vi "VI Tree.vi"   [LabVIEW 2015, in "Keithley 2450.lvlib"]
doc: "This is the instrument driver for the Keithley 2400 Series SourceMeter. The VI Tree displays all the user-callable VIs of the instrument driver in an organized table."
uses:
  <instrlib>/Keithley 2450/Keithley 2450.lvlib
panel:
  # "SEE DIAGRAM\nFOR VI TREE."
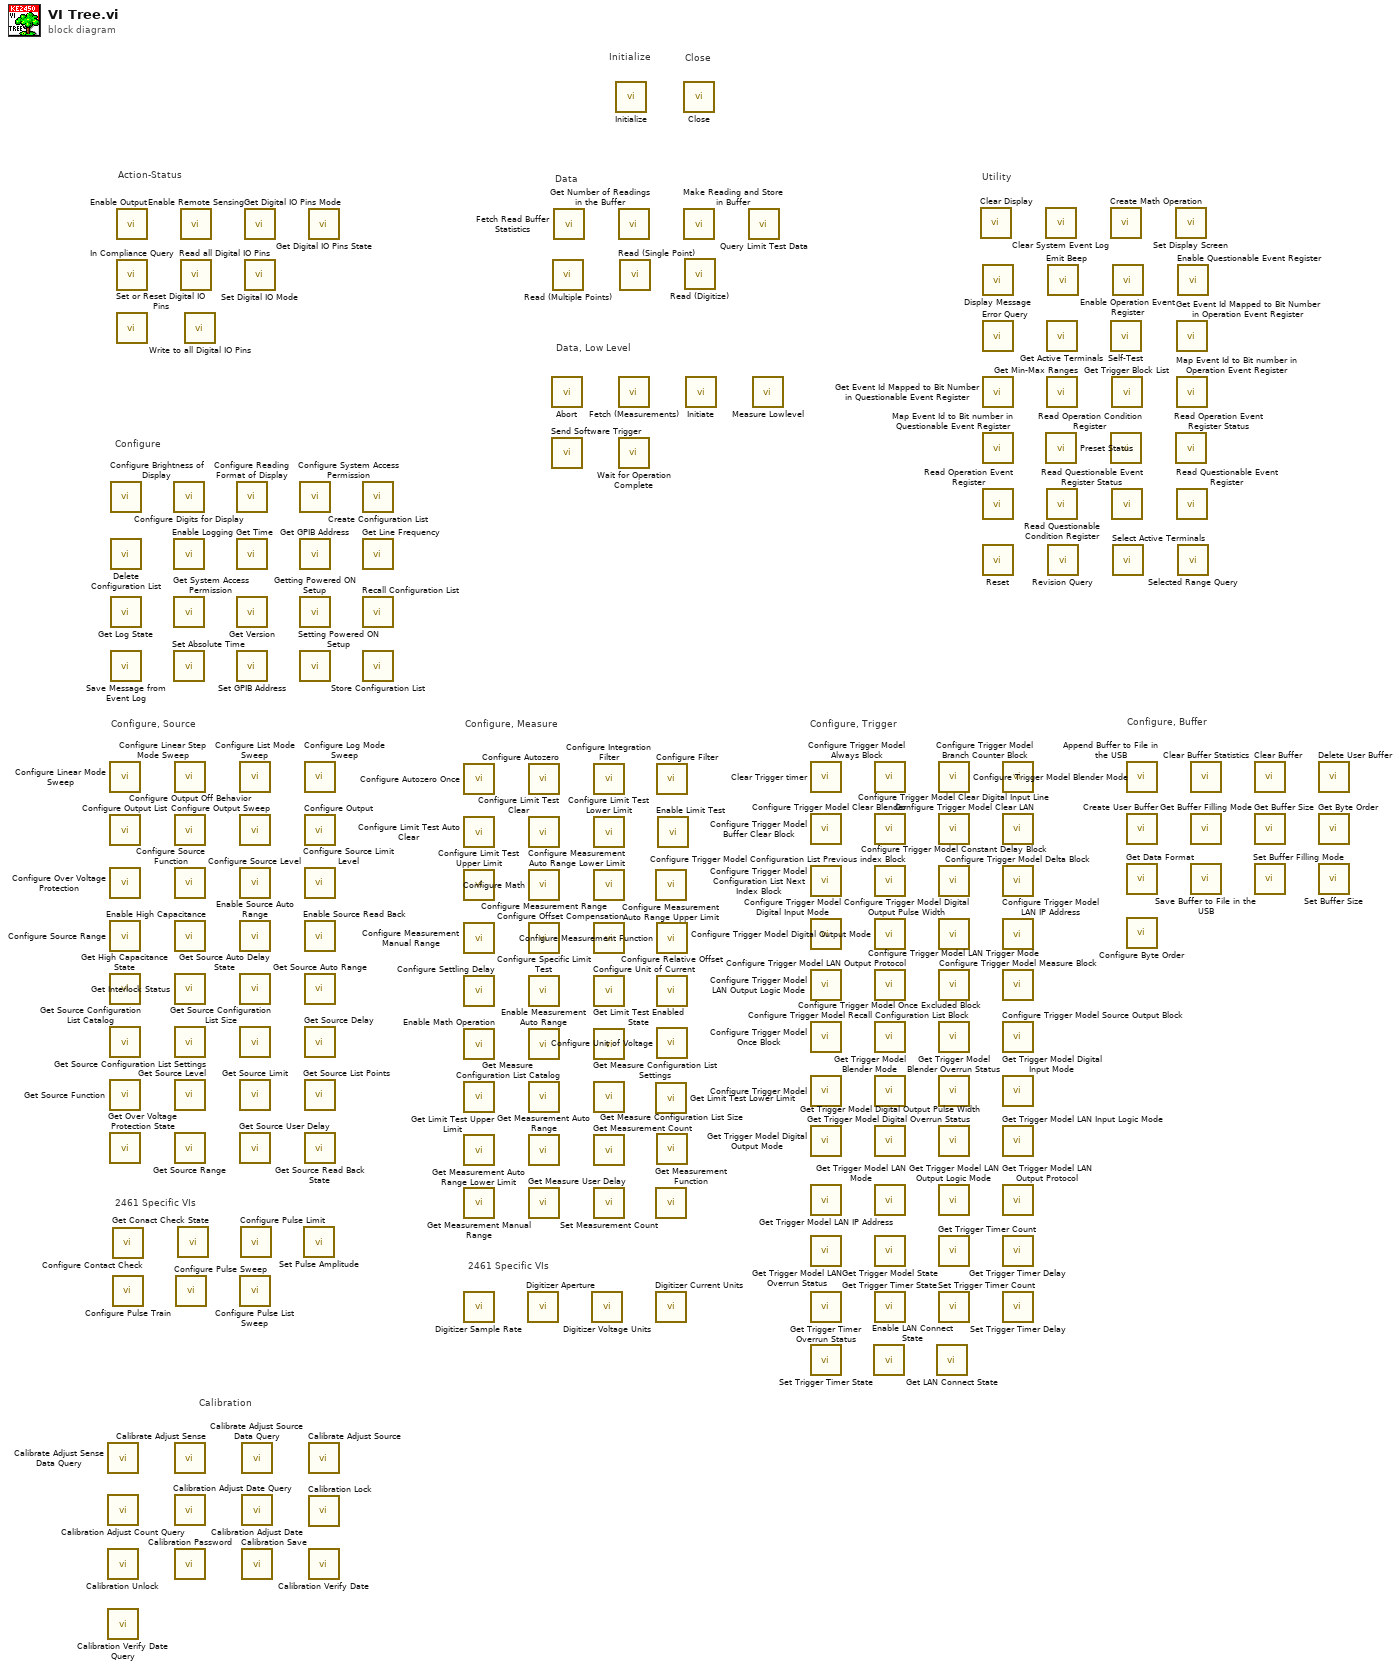
[diagram p0: block diagram]
diagram:
  # "2461 Specific VIs"
  # "Calibration"
  # "2461 Specific VIs"
  # "Configure, Buffer"
  # "Configure, Trigger"
  # "Configure, Measure"
  # "Configure, Source"
  # "Configure"
  # "Utility"
  # "Data, Low Level"
  # "Data"
  # "Action-Status"
  # "Close"
  # "Initialize"
  n1 = call <instrlib>:"Calibrate Adjust Sense Data Query.vi"() -> ()  [unwired: 9 in, 3 out]
  n2 = call <instrlib>:"Calibration Adjust Count Query.vi"() -> ()  [unwired: 9 in, 3 out]
  n3 = call <instrlib>:"Calibration Unlock.vi"() -> ()  [unwired: 10 in, 2 out]
  n4 = call <instrlib>:"Calibration Verify Date Query.vi"() -> ()  [unwired: 9 in, 3 out]
  n5 = call <instrlib>:"Configure Linear Mode Sweep.vi"() -> ()  [unwired: 18 in, 2 out]
  n6 = call <instrlib>:"Configure Output List.vi"() -> ()  [unwired: 10 in, 2 out]
  n7 = call <instrlib>:"Configure Over Voltage Protection.vi"() -> ()  [unwired: 10 in, 2 out]
  n8 = call <instrlib>:"Configure Source Range.vi"() -> ()  [unwired: 10 in, 2 out]
  n9 = call <instrlib>:"Get High Capacitance State.vi"() -> ()  [unwired: 8 in, 4 out]
  n10 = call <instrlib>:"Get Source Configuration List Catalog.vi"() -> ()  [unwired: 9 in, 3 out]
  n11 = call <instrlib>:"Get Source Function.vi"() -> ()  [unwired: 9 in, 3 out]
  n12 = call <instrlib>:"Get Over Voltage Protection State.vi"() -> ()  [unwired: 9 in, 3 out]
  n13 = call <instrlib>:"Configure Brightness of Display.vi"() -> ()  [unwired: 10 in, 2 out]
  n14 = call <instrlib>:"Delete Configuration List.vi"() -> ()  [unwired: 18 in, 2 out]
  n15 = call <instrlib>:"Get Log State.vi"() -> ()  [unwired: 9 in, 3 out]
  n16 = call <instrlib>:"Save Message from Event Log.vi"() -> ()  [unwired: 10 in, 2 out]
  n17 = call <instrlib>:"Configure Contact Check.vi"() -> ()  [unwired: 10 in, 2 out]
  n18 = call <instrlib>:"Configure Pulse Train.vi"() -> ()  [unwired: 18 in, 2 out]
  n19 = call <instrlib>:"Enable Output.vi"() -> ()  [unwired: 10 in, 2 out]
  n20 = call <instrlib>:"In Compliance Query.vi"() -> ()  [unwired: 8 in, 4 out]
  n21 = call <instrlib>:"Set or Reset Digital IO Pins.vi"() -> ()  [unwired: 10 in, 2 out]
  n22 = call <instrlib>:"Configure Digits for Display.vi"() -> ()  [unwired: 10 in, 2 out]
  n23 = call <instrlib>:"Enable Logging.vi"() -> ()  [unwired: 10 in, 2 out]
  n24 = call <instrlib>:"Get System Access Permission.vi"() -> ()  [unwired: 9 in, 3 out]
  n25 = call <instrlib>:"Set Absolute Time.vi"() -> ()  [unwired: 10 in, 2 out]
  n26 = call <instrlib>:"Configure Linear Step Mode Sweep.vi"() -> ()  [unwired: 18 in, 2 out]
  n27 = call <instrlib>:"Configure Output Off Behavior.vi"() -> ()  [unwired: 10 in, 2 out]
  n28 = call <instrlib>:"Configure Source Function.vi"() -> ()  [unwired: 10 in, 2 out]
  n29 = call <instrlib>:"Enable High Capacitance.vi"() -> ()  [unwired: 10 in, 2 out]
  n30 = call <instrlib>:"Get Interlock Status.vi"() -> ()  [unwired: 9 in, 3 out]
  n31 = call <instrlib>:"Get Source Configuration List Settings.vi"() -> ()  [unwired: 17 in, 3 out]
  n32 = call <instrlib>:"Get Source Level.vi"() -> ()  [unwired: 8 in, 4 out]
  n33 = call <instrlib>:"Get Source Range.vi"() -> ()  [unwired: 8 in, 4 out]
  n34 = call <instrlib>:"Calibrate Adjust Sense.vi"() -> ()  [unwired: 10 in, 2 out]
  n35 = call <instrlib>:"Calibration Adjust Date Query.vi"() -> ()  [unwired: 9 in, 3 out]
  n36 = call <instrlib>:"Calibration Password.vi"() -> ()  [unwired: 10 in, 2 out]
  n37 = call <instrlib>:"Configure Pulse Sweep.vi"() -> ()  [unwired: 18 in, 2 out]
  n38 = call <instrlib>:"Get Conact Check State.vi"() -> ()  [unwired: 6 in, 6 out]
  n39 = call <instrlib>:"Enable Remote Sensing.vi"() -> ()  [unwired: 10 in, 2 out]
  n40 = call <instrlib>:"Read all Digital IO Pins.vi"() -> ()  [unwired: 9 in, 3 out]
  n41 = call <instrlib>:"Write to all Digital IO Pins.vi"() -> ()  [unwired: 10 in, 2 out]
  n42 = call <instrlib>:"Configure Reading Format of Display.vi"() -> ()  [unwired: 10 in, 2 out]
  n43 = call <instrlib>:"Get Time.vi"() -> ()  [unwired: 8 in, 4 out]
  n44 = call <instrlib>:"Get Version.vi"() -> ()  [unwired: 9 in, 3 out]
  n45 = call <instrlib>:"Set GPIB Address.vi"() -> ()  [unwired: 10 in, 2 out]
  n46 = call <instrlib>:"Configure List Mode Sweep.vi"() -> ()  [unwired: 14 in, 2 out]
  n47 = call <instrlib>:"Configure Output Sweep.vi"() -> ()  [unwired: 14 in, 2 out]
  n48 = call <instrlib>:"Configure Source Level.vi"() -> ()  [unwired: 10 in, 2 out]
  n49 = call <instrlib>:"Enable Source Auto Range.vi"() -> ()  [unwired: 10 in, 2 out]
  n50 = call <instrlib>:"Get Source Auto Delay State.vi"() -> ()  [unwired: 9 in, 3 out]
  n51 = call <instrlib>:"Get Source Configuration List Size.vi"() -> ()  [unwired: 9 in, 3 out]
  n52 = call <instrlib>:"Get Source Limit.vi"() -> ()  [unwired: 8 in, 4 out]
  n53 = call <instrlib>:"Get Source User Delay.vi"() -> ()  [unwired: 9 in, 3 out]
  n54 = call <instrlib>:"Configure Pulse List Sweep.vi"() -> ()  [unwired: 18 in, 2 out]
  n55 = call <instrlib>:"Configure Pulse Limit.vi"() -> ()  [unwired: 10 in, 2 out]
  n56 = call <instrlib>:"Calibrate Adjust Source Data Query.vi"() -> ()  [unwired: 9 in, 3 out]
  n57 = call <instrlib>:"Calibration Adjust Date.vi"() -> ()  [unwired: 10 in, 2 out]
  n58 = call <instrlib>:"Calibration Save.vi"() -> ()  [unwired: 10 in, 2 out]
  n59 = call <instrlib>:"Get Digital IO Pins Mode.vi"() -> ()  [unwired: 9 in, 3 out]
  n60 = call <instrlib>:"Set Digital IO Mode.vi"() -> ()  [unwired: 10 in, 2 out]
  n61 = call <instrlib>:"Configure System Access Permission.vi"() -> ()  [unwired: 10 in, 2 out]
  n62 = call <instrlib>:"Get GPIB Address.vi"() -> ()  [unwired: 9 in, 3 out]
  n63 = call <instrlib>:"Getting Powered ON Setup.vi"() -> ()  [unwired: 9 in, 3 out]
  n64 = call <instrlib>:"Setting Powered ON Setup.vi"() -> ()  [unwired: 10 in, 2 out]
  n65 = call <instrlib>:"Set Pulse Amplitude.vi"() -> ()  [unwired: 10 in, 2 out]
  n66 = call <instrlib>:"Configure Log Mode Sweep.vi"() -> ()  [unwired: 18 in, 2 out]
  n67 = call <instrlib>:"Configure Output.vi"() -> ()  [unwired: 14 in, 2 out]
  n68 = call <instrlib>:"Configure Source Limit Level.vi"() -> ()  [unwired: 10 in, 2 out]
  n69 = call <instrlib>:"Enable Source Read Back.vi"() -> ()  [unwired: 10 in, 2 out]
  n70 = call <instrlib>:"Get Source Auto Range.vi"() -> ()  [unwired: 8 in, 4 out]
  n71 = call <instrlib>:"Get Source Delay.vi"() -> ()  [unwired: 9 in, 3 out]
  n72 = call <instrlib>:"Get Source List Points.vi"() -> ()  [unwired: 8 in, 4 out]
  n73 = call <instrlib>:"Get Source Read Back State.vi"() -> ()  [unwired: 8 in, 4 out]
  n74 = call <instrlib>:"Get Digital IO Pins State.vi"() -> ()  [unwired: 9 in, 3 out]
  n75 = call <instrlib>:"Calibrate Adjust Source.vi"() -> ()  [unwired: 10 in, 2 out]
  n76 = call <instrlib>:"Calibration Lock.vi"() -> ()  [unwired: 10 in, 2 out]
  n77 = call <instrlib>:"Calibration Verify Date.vi"() -> ()  [unwired: 10 in, 2 out]
  n78 = call <instrlib>:"Create Configuration List.vi"() -> ()  [unwired: 10 in, 2 out]
  n79 = call <instrlib>:"Get Line Frequency.vi"() -> ()  [unwired: 9 in, 3 out]
  n80 = call <instrlib>:"Recall Configuration List.vi"() -> ()  [unwired: 18 in, 2 out]
  n81 = call <instrlib>:"Store Configuration List.vi"() -> ()  [unwired: 18 in, 2 out]
  n82 = call <instrlib>:"Configure Autozero Once.vi"() -> ()  [unwired: 10 in, 2 out]
  n83 = call <instrlib>:"Configure Limit Test Auto Clear.vi"() -> ()  [unwired: 14 in, 2 out]
  n84 = call <instrlib>:"Configure Limit Test Upper Limit.vi"() -> ()  [unwired: 14 in, 2 out]
  n85 = call <instrlib>:"Configure Measurement Manual Range.vi"() -> ()  [unwired: 10 in, 2 out]
  n86 = call <instrlib>:"Configure Settling Delay.vi"() -> ()  [unwired: 10 in, 2 out]
  n87 = call <instrlib>:"Enable Math Operation.vi"() -> ()  [unwired: 10 in, 2 out]
  n88 = call <instrlib>:"Get Limit Test Upper Limit.vi"() -> ()  [unwired: 13 in, 3 out]
  n89 = call <instrlib>:"Get Measurement Auto Range Lower Limit.vi"() -> ()  [unwired: 11 in, 5 out]
  n90 = call <instrlib>:"Get Measurement Manual Range.vi"() -> ()  [unwired: 11 in, 5 out]
  n91 = call <instrlib>:"Digitizer Sample Rate.vi"() -> ()  [unwired: 10 in, 2 out]
  n92 = call <instrlib>:"Digitizer Aperture.vi"() -> ()  [unwired: 14 in, 2 out]
  n93 = call <instrlib>:"Configure Autozero.vi"() -> ()  [unwired: 10 in, 2 out]
  n94 = call <instrlib>:"Configure Limit Test Clear.vi"() -> ()  [unwired: 14 in, 2 out]
  n95 = call <instrlib>:"Configure Math.vi"() -> ()  [unwired: 18 in, 2 out]
  n96 = call <instrlib>:"Configure Measurement Range.vi"() -> ()  [unwired: 10 in, 2 out]
  n97 = call <instrlib>:"Configure Specific Limit Test.vi"() -> ()  [unwired: 14 in, 2 out]
  n98 = call <instrlib>:"Enable Measurement Auto Range.vi"() -> ()  [unwired: 10 in, 2 out]
  n99 = call <instrlib>:"Get Measure Configuration List Catalog.vi"() -> ()  [unwired: 9 in, 3 out]
  n100 = call <instrlib>:"Get Measurement Auto Range.vi"() -> ()  [unwired: 11 in, 5 out]
  n101 = call <instrlib>:"Get Measure User Delay.vi"() -> ()  [unwired: 9 in, 3 out]
  n102 = call <instrlib>:"Abort.vi"() -> ()  [unwired: 10 in, 2 out]
  n103 = call <instrlib>:"Send Software Trigger.vi"() -> ()  [unwired: 10 in, 2 out]
  n104 = call <instrlib>:"Read (Multiple Points).vi"() -> ()  [unwired: 13 in, 3 out]
  n105 = call <instrlib>:"Fetch Read Buffer Statistics.vi"() -> ()  [unwired: 13 in, 3 out]
  n106 = call <instrlib>:"Digitizer Voltage Units.vi"() -> ()  [unwired: 10 in, 2 out]
  n107 = call <instrlib>:"Configure Integration Filter.vi"() -> ()  [unwired: 10 in, 2 out]
  n108 = call <instrlib>:"Configure Limit Test Lower Limit.vi"() -> ()  [unwired: 14 in, 2 out]
  n109 = call <instrlib>:"Configure Measurement Auto Range Lower Limit.vi"() -> ()  [unwired: 10 in, 2 out]
  n110 = call <instrlib>:"Configure Offset Compensation.vi"() -> ()  [unwired: 10 in, 2 out]
  n111 = call <instrlib>:"Configure Unit of Current.vi"() -> ()  [unwired: 10 in, 2 out]
  n112 = call <instrlib>:"Get Limit Test Enabled State.vi"() -> ()  [unwired: 13 in, 3 out]
  n113 = call <instrlib>:"Get Measure Configuration List Settings.vi"() -> ()  [unwired: 17 in, 3 out]
  n114 = call <instrlib>:"Get Measurement Count.vi"() -> ()  [unwired: 9 in, 3 out]
  n115 = call <instrlib>:"Set Measurement Count.vi"() -> ()  [unwired: 10 in, 2 out]
  n116 = call <instrlib>:"Initialize.vi"() -> ()  [unwired: 10 in, 2 out]
  n117 = call <instrlib>:"Get Number of Readings in the Buffer.vi"() -> ()  [unwired: 13 in, 3 out]
  n118 = call <instrlib>:"Fetch (Measurements).vi"() -> ()  [unwired: 13 in, 3 out]
  n119 = call <instrlib>:"Wait for Operation Complete.vi"() -> ()  [unwired: 10 in, 2 out]
  n120 = call <instrlib>:"Read (Single Point).vi"() -> ()  [unwired: 13 in, 3 out]
  n121 = call <instrlib>:"Configure Measurement Auto Range Upper Limit.vi"() -> ()  [unwired: 10 in, 2 out]
  n122 = call <instrlib>:"Get Limit Test Lower Limit.vi"() -> ()  [unwired: 13 in, 3 out]
  n123 = call <instrlib>:"Get Measurement Function.vi"() -> ()  [unwired: 9 in, 3 out]
  n124 = call <instrlib>:"Digitizer Current Units.vi"() -> ()  [unwired: 10 in, 2 out]
  n125 = call <instrlib>:"Configure Filter.vi"() -> ()  [unwired: 18 in, 2 out]
  n126 = call <instrlib>:"Configure Measurement Function.vi"() -> ()  [unwired: 10 in, 2 out]
  n127 = call <instrlib>:"Configure Relative Offset.vi"() -> ()  [unwired: 10 in, 2 out]
  n128 = call <instrlib>:"Configure Unit of Voltage.vi"() -> ()  [unwired: 10 in, 2 out]
  n129 = call <instrlib>:"Get Measure Configuration List Size.vi"() -> ()  [unwired: 9 in, 3 out]
  n130 = call <instrlib>:"Enable Limit Test.vi"() -> ()  [unwired: 14 in, 2 out]
  n131 = call <instrlib>:"Close.vi"() -> ()  [unwired: 11 in, 1 out]
  n132 = call <instrlib>:"Make Reading and Store in Buffer.vi"() -> ()  [unwired: 14 in, 2 out]
  n133 = call <instrlib>:"Read (Digitize).vi"() -> ()  [unwired: 13 in, 3 out]
  n134 = call <instrlib>:"Initiate.vi"() -> ()  [unwired: 10 in, 2 out]
  n135 = call <instrlib>:"Query Limit Test Data.vi"() -> ()  [unwired: 8 in, 4 out]
  n136 = call <instrlib>:"Measure Lowlevel.vi"() -> ()  [unwired: 13 in, 3 out]
  n137 = call <instrlib>:"Clear Trigger timer.vi"() -> ()  [unwired: 10 in, 2 out]
  n138 = call <instrlib>:"Configure Trigger Model Buffer Clear Block.vi"() -> ()  [unwired: 10 in, 2 out]
  n139 = call <instrlib>:"Configure Trigger Model Configuration List Next Index Block.vi"() -> ()  [unwired: 10 in, 2 out]
  n140 = call <instrlib>:"Configure Trigger Model Digital Input Mode.vi"() -> ()  [unwired: 10 in, 2 out]
  n141 = call <instrlib>:"Configure Trigger Model LAN Output Logic Mode.vi"() -> ()  [unwired: 10 in, 2 out]
  n142 = call <instrlib>:"Configure Trigger Model Once Block.vi"() -> ()  [unwired: 10 in, 2 out]
  n143 = call <instrlib>:"Configure Trigger Model.vi"() -> ()  [unwired: 18 in, 2 out]
  n144 = call <instrlib>:"Get Trigger Model Digital Output Mode.vi"() -> ()  [unwired: 9 in, 3 out]
  n145 = call <instrlib>:"Get Trigger Model LAN IP Address.vi"() -> ()  [unwired: 9 in, 3 out]
  n146 = call <instrlib>:"Get Trigger Model LAN Overrun Status.vi"() -> ()  [unwired: 9 in, 3 out]
  n147 = call <instrlib>:"Get Trigger Timer Overrun Status.vi"() -> ()  [unwired: 9 in, 3 out]
  n148 = call <instrlib>:"Set Trigger Timer State.vi"() -> ()  [unwired: 10 in, 2 out]
  n149 = call <instrlib>:"Enable LAN Connect State.vi"() -> ()  [unwired: 10 in, 2 out]
  n150 = call <instrlib>:"Configure Trigger Model Always Block.vi"() -> ()  [unwired: 10 in, 2 out]
  n151 = call <instrlib>:"Configure Trigger Model Clear Blender.vi"() -> ()  [unwired: 10 in, 2 out]
  n152 = call <instrlib>:"Configure Trigger Model Configuration List Previous index Block.vi"() -> ()  [unwired: 10 in, 2 out]
  n153 = call <instrlib>:"Configure Trigger Model Digital Output Mode.vi"() -> ()  [unwired: 10 in, 2 out]
  n154 = call <instrlib>:"Configure Trigger Model LAN Output Protocol.vi"() -> ()  [unwired: 10 in, 2 out]
  n155 = call <instrlib>:"Configure Trigger Model Once Excluded Block.vi"() -> ()  [unwired: 10 in, 2 out]
  n156 = call <instrlib>:"Get Trigger Model Blender Mode.vi"() -> ()  [unwired: 9 in, 3 out]
  n157 = call <instrlib>:"Get Trigger Model Digital Output Pulse Width.vi"() -> ()  [unwired: 9 in, 3 out]
  n158 = call <instrlib>:"Get Trigger Model LAN Mode.vi"() -> ()  [unwired: 9 in, 3 out]
  n159 = call <instrlib>:"Get Trigger Model State.vi"() -> ()  [unwired: 8 in, 4 out]
  n160 = call <instrlib>:"Get Trigger Timer State.vi"() -> ()  [unwired: 9 in, 3 out]
  n161 = call <instrlib>:"Get LAN Connect State.vi"() -> ()  [unwired: 9 in, 3 out]
  n162 = call <instrlib>:"Configure Trigger Model Blender Mode.vi"() -> ()  [unwired: 10 in, 2 out]
  n163 = call <instrlib>:"Configure Trigger Model Clear Digital Input Line.vi"() -> ()  [unwired: 10 in, 2 out]
  n164 = call <instrlib>:"Configure Trigger Model Constant Delay Block.vi"() -> ()  [unwired: 10 in, 2 out]
  n165 = call <instrlib>:"Configure Trigger Model Digital Output Pulse Width.vi"() -> ()  [unwired: 10 in, 2 out]
  n166 = call <instrlib>:"Configure Trigger Model LAN Trigger Mode.vi"() -> ()  [unwired: 10 in, 2 out]
  n167 = call <instrlib>:"Configure Trigger Model Recall Configuration List Block.vi"() -> ()  [unwired: 18 in, 2 out]
  n168 = call <instrlib>:"Get Trigger Model Blender Overrun Status.vi"() -> ()  [unwired: 9 in, 3 out]
  n169 = call <instrlib>:"Get Trigger Model Digital Overrun Status.vi"() -> ()  [unwired: 9 in, 3 out]
  n170 = call <instrlib>:"Get Trigger Model LAN Output Logic Mode.vi"() -> ()  [unwired: 9 in, 3 out]
  n171 = call <instrlib>:"Get Trigger Timer Count.vi"() -> ()  [unwired: 9 in, 3 out]
  n172 = call <instrlib>:"Set Trigger Timer Count.vi"() -> ()  [unwired: 10 in, 2 out]
  n173 = call <instrlib>:"Clear Display.vi"() -> ()  [unwired: 10 in, 2 out]
  n174 = call <instrlib>:"Display Message.vi"() -> ()  [unwired: 10 in, 2 out]
  n175 = call <instrlib>:"Error Query.vi"() -> ()  [unwired: 8 in, 4 out]
  n176 = call <instrlib>:"Get Event Id Mapped to Bit Number in Questionable Event Register.vi"() -> ()  [unwired: 8 in, 4 out]
  n177 = call <instrlib>:"Map Event Id to Bit number in Questionable Event Register.vi"() -> ()  [unwired: 10 in, 2 out]
  n178 = call <instrlib>:"Read Operation Event Register.vi"() -> ()  [unwired: 9 in, 3 out]
  n179 = call <instrlib>:"Reset.vi"() -> ()  [unwired: 10 in, 2 out]
  n180 = call <instrlib>:"Configure Trigger Model Branch Counter Block.vi"() -> ()  [unwired: 14 in, 2 out]
  n181 = call <instrlib>:"Configure Trigger Model Clear LAN.vi"() -> ()  [unwired: 10 in, 2 out]
  n182 = call <instrlib>:"Configure Trigger Model Delta Block.vi"() -> ()  [unwired: 18 in, 2 out]
  n183 = call <instrlib>:"Configure Trigger Model LAN IP Address.vi"() -> ()  [unwired: 10 in, 2 out]
  n184 = call <instrlib>:"Configure Trigger Model Measure Block.vi"() -> ()  [unwired: 10 in, 2 out]
  n185 = call <instrlib>:"Configure Trigger Model Source Output Block.vi"() -> ()  [unwired: 10 in, 2 out]
  n186 = call <instrlib>:"Get Trigger Model Digital Input Mode.vi"() -> ()  [unwired: 9 in, 3 out]
  n187 = call <instrlib>:"Get Trigger Model LAN Input Logic Mode.vi"() -> ()  [unwired: 9 in, 3 out]
  n188 = call <instrlib>:"Get Trigger Model LAN Output Protocol.vi"() -> ()  [unwired: 9 in, 3 out]
  n189 = call <instrlib>:"Get Trigger Timer Delay.vi"() -> ()  [unwired: 9 in, 3 out]
  n190 = call <instrlib>:"Set Trigger Timer Delay.vi"() -> ()  [unwired: 10 in, 2 out]
  n191 = call <instrlib>:"Clear System Event Log.vi"() -> ()  [unwired: 10 in, 2 out]
  n192 = call <instrlib>:"Preset Status.vi"() -> ()  [unwired: 10 in, 2 out]
  n193 = call <instrlib>:"Get Active Terminals.vi"() -> ()  [unwired: 9 in, 3 out]
  n194 = call <instrlib>:"Get Min-Max Ranges.vi"() -> ()  [unwired: 6 in, 6 out]
  n195 = call <instrlib>:"Read Questionable Condition Register.vi"() -> ()  [unwired: 9 in, 3 out]
  n196 = call <instrlib>:"Emit Beep.vi"() -> ()  [unwired: 10 in, 2 out]
  n197 = call <instrlib>:"Revision Query.vi"() -> ()  [unwired: 8 in, 4 out]
  n198 = call <instrlib>:"Create Math Operation.vi"() -> ()  [unwired: 18 in, 2 out]
  n199 = call <instrlib>:"Self-Test.vi"() -> ()  [unwired: 8 in, 4 out]
  n200 = call <instrlib>:"Read Operation Condition Register.vi"() -> ()  [unwired: 9 in, 3 out]
  n201 = call <instrlib>:"Get Trigger Block List.vi"() -> ()  [unwired: 9 in, 3 out]
  n202 = call <instrlib>:"Read Questionable Event Register Status.vi"() -> ()  [unwired: 9 in, 3 out]
  n203 = call <instrlib>:"Enable Operation Event Register.vi"() -> ()  [unwired: 10 in, 2 out]
  n204 = call <instrlib>:"Select Active Terminals.vi"() -> ()  [unwired: 10 in, 2 out]
  n205 = call <instrlib>:"Append Buffer to File in the USB.vi"() -> ()  [unwired: 14 in, 2 out]
  n206 = call <instrlib>:"Create User Buffer.vi"() -> ()  [unwired: 14 in, 2 out]
  n207 = call <instrlib>:"Get Data Format.vi"() -> ()  [unwired: 13 in, 3 out]
  n208 = call <instrlib>:"Configure Byte Order.vi"() -> ()  [unwired: 14 in, 2 out]
  n209 = call <instrlib>:"Set Display Screen.vi"() -> ()  [unwired: 10 in, 2 out]
  n210 = call <instrlib>:"Read Operation Event Register Status.vi"() -> ()  [unwired: 9 in, 3 out]
  n211 = call <instrlib>:"Get Event Id Mapped to Bit Number in Operation Event Register.vi"() -> ()  [unwired: 8 in, 4 out]
  n212 = call <instrlib>:"Map Event Id to Bit number in Operation Event Register.vi"() -> ()  [unwired: 10 in, 2 out]
  n213 = call <instrlib>:"Read Questionable Event Register.vi"() -> ()  [unwired: 9 in, 3 out]
  n214 = call <instrlib>:"Enable Questionable Event Register.vi"() -> ()  [unwired: 10 in, 2 out]
  n215 = call <instrlib>:"Selected Range Query.vi"() -> ()  [unwired: 9 in, 3 out]
  n216 = call <instrlib>:"Clear Buffer Statistics.vi"() -> ()  [unwired: 14 in, 2 out]
  n217 = call <instrlib>:"Get Buffer Filling Mode.vi"() -> ()  [unwired: 13 in, 3 out]
  n218 = call <instrlib>:"Save Buffer to File in the USB.vi"() -> ()  [unwired: 14 in, 2 out]
  n219 = call <instrlib>:"Clear Buffer.vi"() -> ()  [unwired: 14 in, 2 out]
  n220 = call <instrlib>:"Get Buffer Size.vi"() -> ()  [unwired: 13 in, 3 out]
  n221 = call <instrlib>:"Set Buffer Filling Mode.vi"() -> ()  [unwired: 14 in, 2 out]
  n222 = call <instrlib>:"Delete User Buffer.vi"() -> ()  [unwired: 14 in, 2 out]
  n223 = call <instrlib>:"Get Byte Order.vi"() -> ()  [unwired: 13 in, 3 out]
  n224 = call <instrlib>:"Set Buffer Size.vi"() -> ()  [unwired: 14 in, 2 out]
